vi "Execution Flow.vi"   [LabVIEW 2020]
uses:
  File Type Interface.lvclass
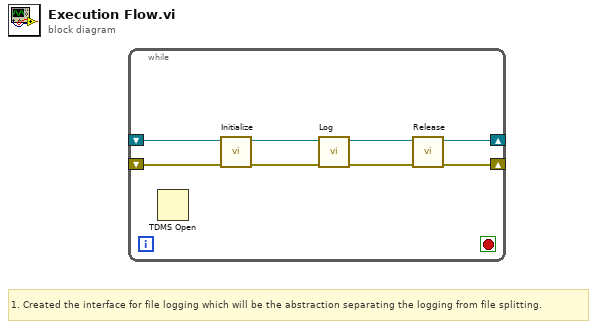
[diagram p0: block diagram]
diagram:
  # "1. Created the interface for file logging which will be the abstraction separating the logging from file splitting."
  n1 = while {
    shift-right: [w4] -> _
    shift-left: _ -> [w3]
    shift-right: [w2] -> _
    shift-left: _ -> [w1]
    stop <- _ stop-if-true
    n2 = TDMS Open() -> ()  [unwired: 7 in, 2 out]
    n3 = call-dynamic "Initialize.vi"("error in"=w1, "File Logger Interface in"=w3) -> ("error out"=w6:errorcluster, "File Logger Interface out"=w5:refnum<class "File Type Interface.lvclass">)  [unwired: 8 in]
    n4 = call-dynamic "Log.vi"("error in"=w6, "File Logger Interface in"=w5) -> ("error out"=w7:errorcluster, "File Logger Interface out"=w8:refnum<class "File Type Interface.lvclass">)  [unwired: 8 in]
    n5 = call-dynamic "Release.vi"("error in"=w7, "File Logger Interface in"=w8) -> ("error out"=w2:errorcluster, "File Logger Interface out"=w4:refnum<class "File Type Interface.lvclass">)  [unwired: 8 in]
  }
